vi "CODMn平行样流程 (子VI).vi"(11 "COD1":bool) -> (3 "布尔":bool)   [LabVIEW 2016, in "质控单元.lvlib"]
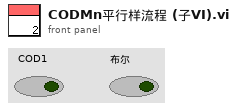
[diagram p1: front panel]
types:
  T1 = enum16{"待机", "启动水样测量", "水样测量中", "启动加标", "启动加标回收", "加标回收测量中", "结束"}
  T2 = cluster{"测量模式":enum16{"水样测量", "标样核查", "零点核查", "跨度核查", "空白测试", "加标回收", "平行样", "校零", "校标"}}
  T3 = cluster{"量程":dbl, "检出限":dbl, "加标前水样浓度":dbl, "加标后水样浓度":dbl, "加标水杯定容体积":dbl, "加标母液浓度":dbl, "加标体积":dbl, "加标回收率":dbl}
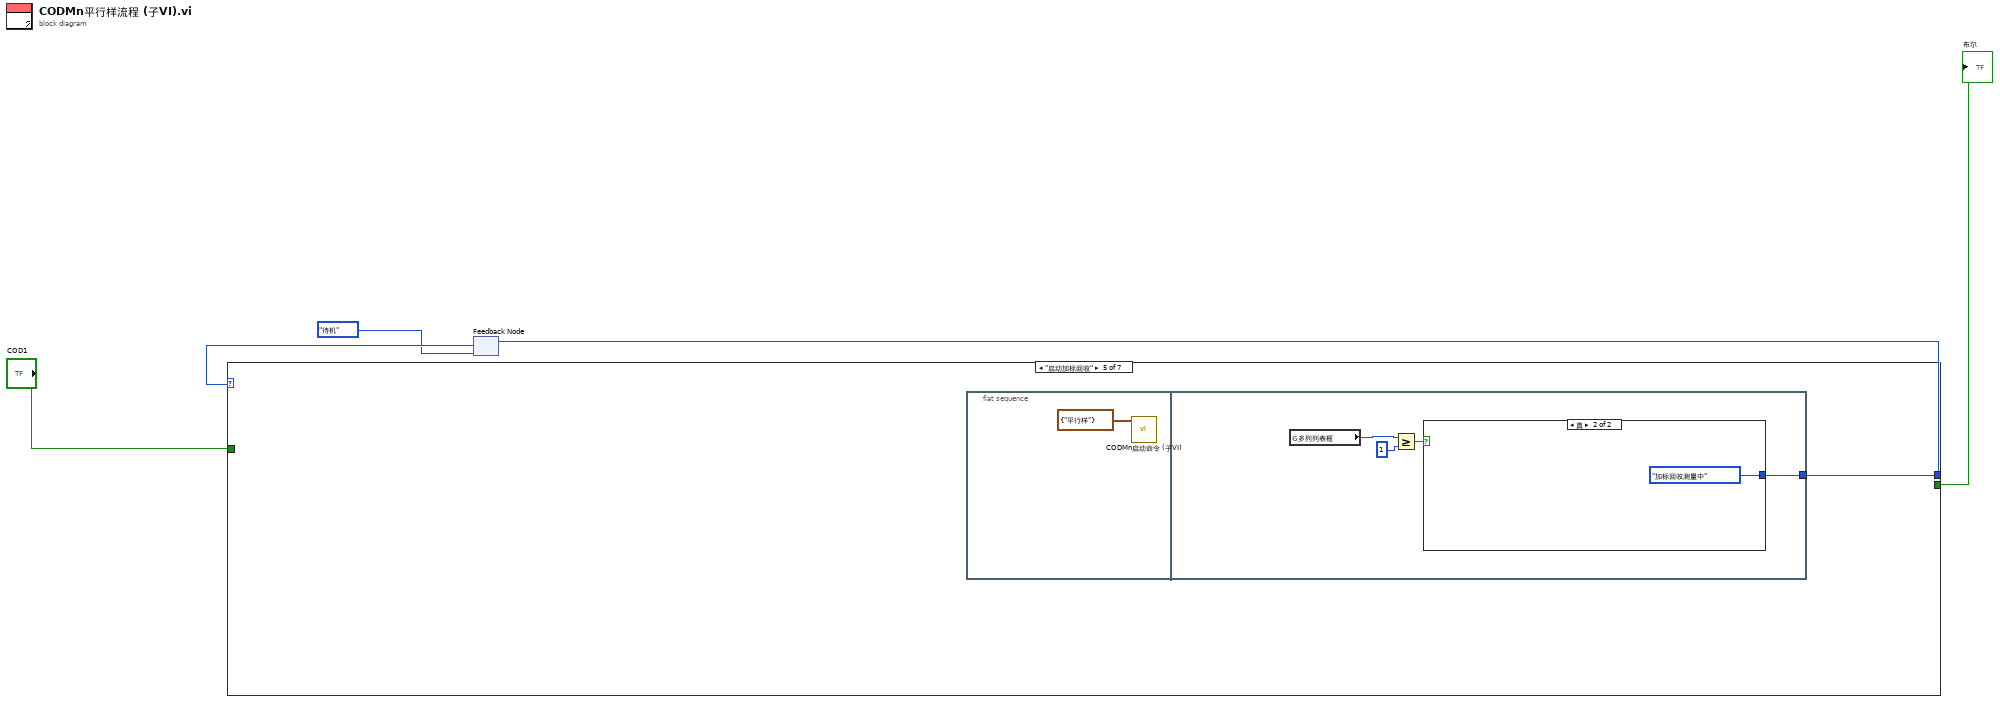
[diagram p0: block diagram]
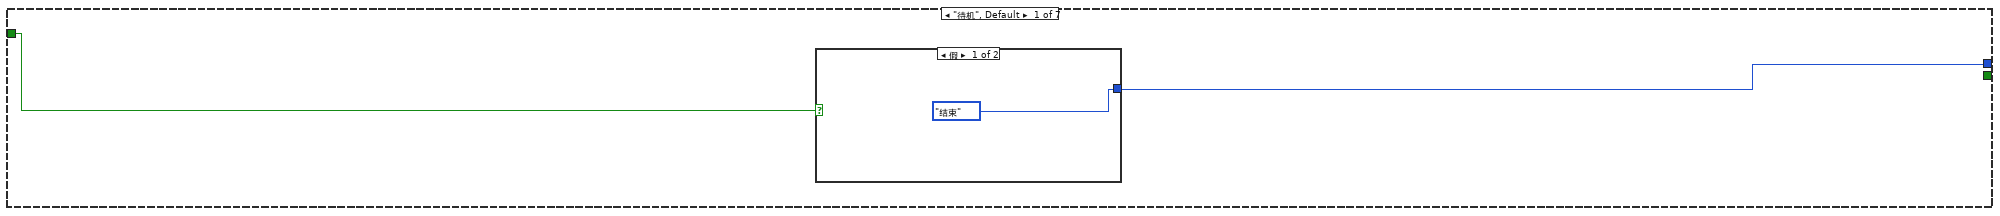
[diagram p2: hidden frame]
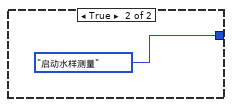
[diagram p3: hidden frame]
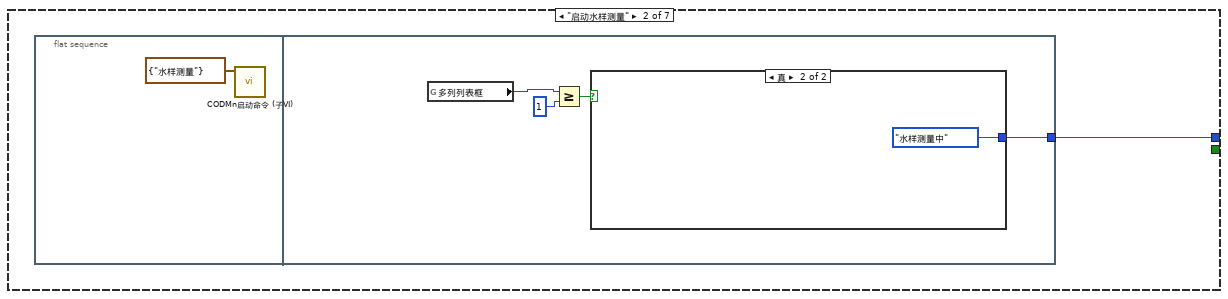
[diagram p4: hidden frame]
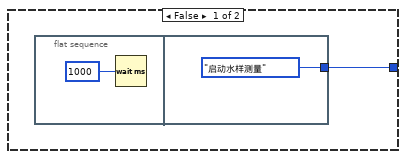
[diagram p5: hidden frame]
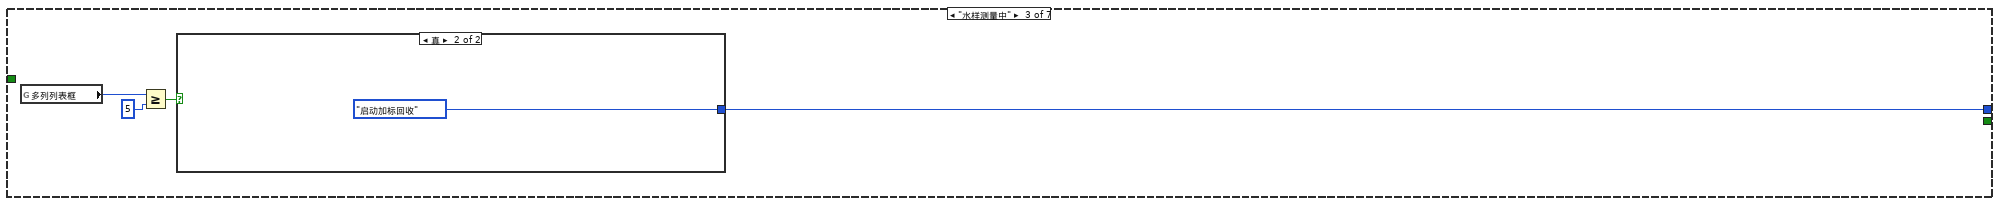
[diagram p6: hidden frame]
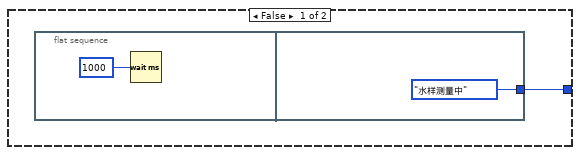
[diagram p7: hidden frame]
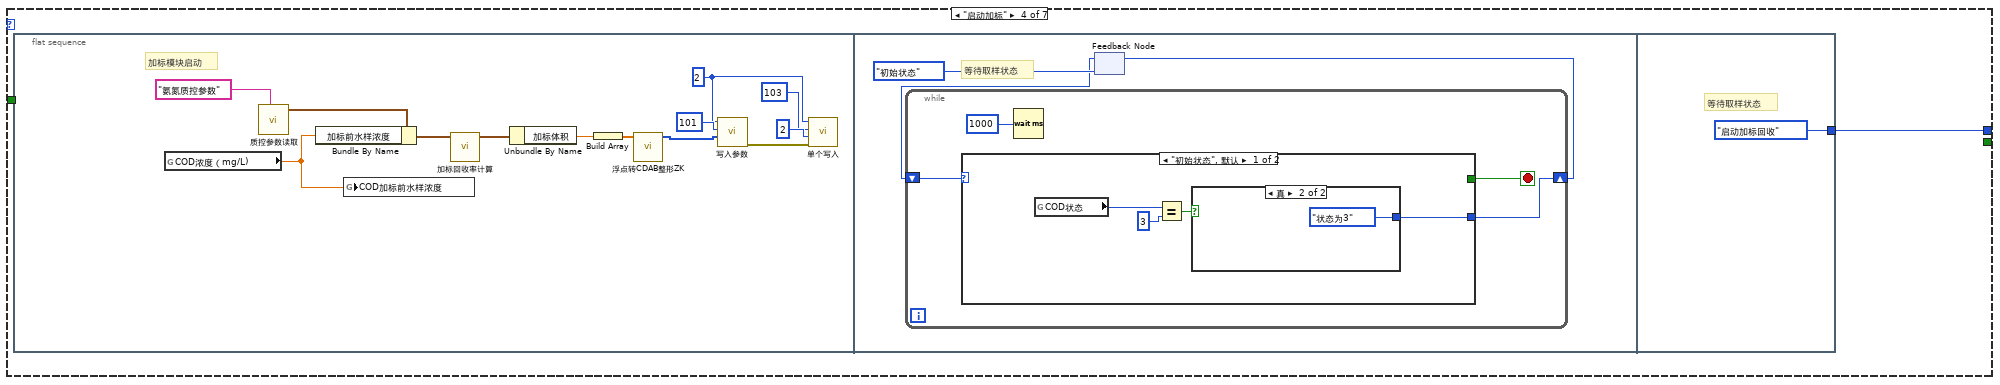
[diagram p8: hidden frame]
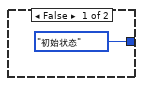
[diagram p9: hidden frame]
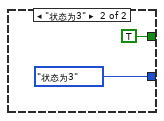
[diagram p10: hidden frame]
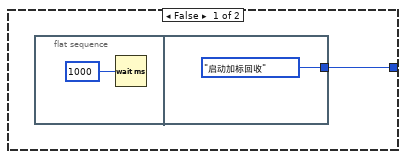
[diagram p11: hidden frame]
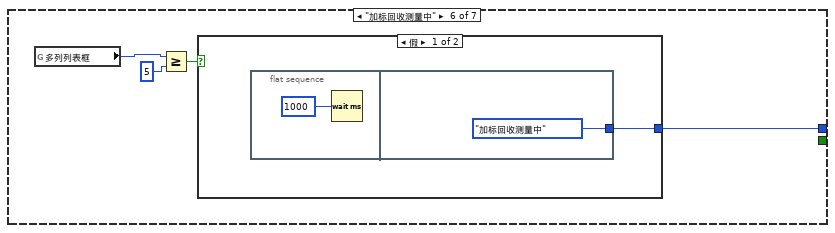
[diagram p12: hidden frame]
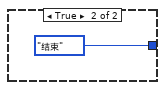
[diagram p13: hidden frame]
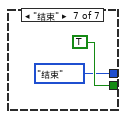
[diagram p14: hidden frame]
diagram:
  n1 = feedback #1(T1."待机") -> (w3:T1)
  n2 = case shown="\"启动加标回收\"" w3 {
    tunnel: [w6 w10 w20 w28 w58 w68 T1."结束"] -> w4
    tunnel: [_ _ _ _ _ _ TRUE] -> w2
    tunnel: "COD1" -> [w7 _ _ _ _ _ _]
    frame "待机", Default {
      n3 = case shown="假" w7 {
        tunnel: [T1."结束" T1."启动水样测量"] -> w6
        frame False {
        }
        frame True {
        }
      }
    }
    frame "启动水样测量" {
      n4 = flat-sequence {
        tunnel: [w12] -> w10
        frame #0 {
          n5 = call "CODMn启动命令 (子VI).vi"("启动测量模式"=T2 {"测量模式"=enum."水样测量"}) -> ()  [unwired: 10 in, 1 out]
        }
        frame #1 {
          n6 = global read "与CODMn交互全局.vi" "多列列表框"() -> (w15:i32)
          n7 = Greater Or Equal?(x=w15, y=1) -> (x >= y?=w14:bool)
          n8 = case shown="真" w14 {
            tunnel: [w16 T1."水样测量中"] -> w12
            frame False {
              n9 = flat-sequence {
                tunnel: [T1."启动水样测量"] -> w16
                frame #0 {
                  n10 = Wait (ms)(milliseconds to wait=u32 1000 ("等待时间（毫秒）")) -> ()  [unwired: 1 out]
                }
                frame #1 {
                }
              }
            }
            frame True {
            }
          }
        }
      }
    }
    frame "水样测量中" {
      n11 = global read "与CODMn交互全局.vi" "多列列表框"() -> (w21:i32)
      n12 = Greater Or Equal?(x=w21, y=5) -> (x >= y?=w22:bool)
      n13 = case shown="真" w22 {
        tunnel: [w24 T1."启动加标回收"] -> w20
        frame False {
          n14 = flat-sequence {
            tunnel: [T1."水样测量中"] -> w24
            frame #0 {
              n15 = Wait (ms)(milliseconds to wait=u32 1000 ("等待时间（毫秒）")) -> ()  [unwired: 1 out]
            }
            frame #1 {
            }
          }
        }
        frame True {
        }
      }
    }
    frame "启动加标" {
      n16 = flat-sequence {
        tunnel: [T1."启动加标回收"] -> w28
        frame #0 {
          w31 = u16 2 ("value")
          # "加标模块启动"
          n17 = global read "与CODMn交互全局.vi" "COD浓度（mg/L)"() -> (w29:dbl)
          n18 = call "质控参数读取.vi"("section"="氨氮质控参数") -> ("参数"=w39:T3)  [unwired: 9 in, 1 out]
          n19 = Bundle By Name(cluster=w39, "加标前水样浓度"=w29) -> (w40:T3)
          n20 = global write "水样浓度全局.vi" "COD加标前水样浓度"(w29) -> ()
          n21 = call "加标回收率计算.vi"("参数"=w40) -> ("参数 out"=w38:T3)  [unwired: 10 in]
          n22 = Unbundle By Name(w38) -> ("加标体积"=w30:dbl)
          n23 = Build Array(w30) -> (w37:dbl[])
          n24 = call "浮点转CDAB整形ZK.vi"("浮点数"=w37) -> ("CDAB整形输出"=w32:u16[])  [unwired: 10 in]
          n25 = call "写入参数.vi"("values"=w32, "starting address"=u16 101, "Slave ID"=w31) -> ("error out"=w36:errorcluster)  [unwired: 8 in]
          n26 = call "单个写入.vi"("Error in"=w36, "value"=u16 2, "address"=u16 103, "Slave ID"=w31) -> ()  [unwired: 7 in, 1 out]
        }
        frame #1 {
          # "等待取样状态"
          n27 = feedback #2(enum16{"初始状态", "状态为3"}."初始状态") -> (w43:enum16{"初始状态", "状态为3"})
          n28 = while {
            shift-right: [w47] -> w42
            shift-left: w43 -> [w48]
            stop <- w46 stop-if-true
            n29 = case shown="\"初始状态\", 默认" w48 {
              tunnel: [w49 enum16{"初始状态", "状态为3"}."状态为3"] -> w47
              tunnel: [_ TRUE] -> w46
              frame "初始状态", Default {
                n30 = global read "加标回收状态全局变量.vi" "COD状态"() -> (w51:u16)
                n31 = Equal?(x=w51, y=u16 3) -> (x = y?=w50:bool)
                n32 = case shown="真" w50 {
                  tunnel: [enum16{"初始状态", "状态为3"}."初始状态" enum16{"初始状态", "状态为3"}."状态为3"] -> w49
                  frame False {
                  }
                  frame True {
                  }
                }
              }
              frame "状态为3" {
              }
            }
            n33 = Wait (ms)(milliseconds to wait=u32 1000 ("等待时间（毫秒）")) -> ()  [unwired: 1 out]
          }
          n34 = feedback-in #2(w42) -> ()
        }
        frame #2 {
          # "等待取样状态"
        }
      }
    }
    frame "启动加标回收" {
      n35 = flat-sequence {
        tunnel: [w60] -> w58
        frame #0 {
          n36 = call "CODMn启动命令 (子VI).vi"("启动测量模式"=T2 {"测量模式"=enum."平行样"}) -> ()  [unwired: 10 in, 1 out]
        }
        frame #1 {
          n37 = global read "与CODMn交互全局.vi" "多列列表框"() -> (w61:i32)
          n38 = Greater Or Equal?(x=w61, y=1) -> (x >= y?=w62:bool)
          n39 = case shown="真" w62 {
            tunnel: [w64 T1."加标回收测量中"] -> w60
            frame False {
              n40 = flat-sequence {
                tunnel: [T1."启动加标回收"] -> w64
                frame #0 {
                  n41 = Wait (ms)(milliseconds to wait=u32 1000 ("等待时间（毫秒）")) -> ()  [unwired: 1 out]
                }
                frame #1 {
                }
              }
            }
            frame True {
            }
          }
        }
      }
    }
    frame "加标回收测量中" {
      n42 = global read "与CODMn交互全局.vi" "多列列表框"() -> (w69:i32)
      n43 = Greater Or Equal?(x=w69, y=5) -> (x >= y?=w70:bool)
      n44 = case shown="假" w70 {
        tunnel: [w72 T1."结束"] -> w68
        frame False {
          n45 = flat-sequence {
            tunnel: [T1."加标回收测量中"] -> w72
            frame #0 {
              n46 = Wait (ms)(milliseconds to wait=u32 1000 ("等待时间（毫秒）")) -> ()  [unwired: 1 out]
            }
            frame #1 {
            }
          }
        }
        frame True {
        }
      }
    }
    frame "结束" {
    }
  }
  "布尔" <- w2
  n47 = feedback-in #1(w4) -> ()
